vi "ChangeBranchName.vi"(10 "New Name":string, 11 "Node In":refnum<data-value>) -> (2 "New Name Out":string, 3 "Node Out":refnum<data-value>)   [LabVIEW 2019]
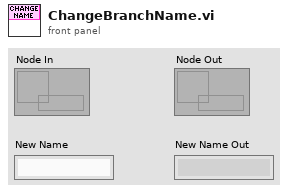
[diagram p1: front panel]
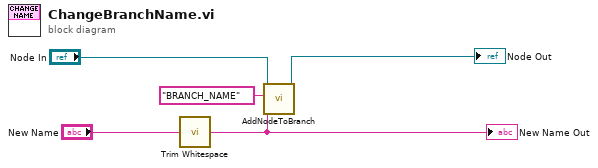
[diagram p0: block diagram]
diagram:
  n1 = call <vilib>:"Trim Whitespace.vi"("string"="New Name") -> ("trimmed string"=w1:string)  [unwired: 1 in]
  "New Name Out" <- w1
  n2 = call "AddNodeToBranch.vi"("Data"=w1, "Unique Node Name"="BRANCH_NAME", "Parent Node In"="Node In") -> ("Parent Node Out"=→"Node Out":refnum<data-value>)  [unwired: 8 in]
